vi "dfd_FXP Lattice ARMA (normalized) with IS.vi"(6 "state in":i64[](array[numeric]), 7 "FXPOPs":T5[](array[typedef]) {"source" items=["Coef a/k"=0, "Coef b/v"=7, "Input"=1, "Output"=2, "Multiplicand"=3, "Product"=4, "Sum"=5, "Delay"=6, "Gain"=8]}, 8 "filtering statistics in":T4(array[cluster]) {"statistics information"."min value" format="%.2f"; "statistics information"."max value" format="%.2f"; "Quantizer Source" items=["Coefficients a/k"=0, "Coefficients b/v"=7, "Input"=1, "Output"=2, "Multiplicand"=3, "Product"=4, "Sum"=5, "Delay"=6]}, 9 "coef v":T7, 10 "coef k & ^k":T7, 11 "X":T7) -> (0 "filtering statistics out":T4(array[cluster]) {"statistics information"."min value" format="%.2f"; "statistics information"."max value" format="%.2f"; "Quantizer Source" items=["Coefficients a/k"=0, "Coefficients b/v"=7, "Input"=1, "Output"=2, "Multiplicand"=3, "Product"=4, "Sum"=5, "Delay"=6]}, 3 "filtered X":T7, 4 "state out":i64[](array[numeric]))   [LabVIEW 2017, in "NI_DigFilter_FXP.lvlib"]
uses:
  <vilib>/addons/Digital Filter Design/NI_DigFilter_FXP.lvlib
  <vilib>/addons/Digital Filter Design/_Objects.llb/dfd_DFXP Data Type (vector).ctl
  <vilib>/addons/Digital Filter Design/_Objects.llb/dfd_DFXP Operation Parameter.ctl
  <vilib>/addons/Digital Filter Design/_Objects.llb/dfd_Internal Quantization Srcs.ctl
  <vilib>/addons/Digital Filter Design/_Objects.llb/DFD Quantization Sources.ctl
  <vilib>/addons/Digital Filter Design/_Objects.llb/DFD FXP Statistics Data.ctl
  <vilib>/addons/Digital Filter Design/_Objects.llb/dfd_DFXP Data Type (scaler).ctl
  <vilib>/addons/Digital Filter Design/NI_DigFilterLicensed.lvlib
panel:
  in  "DFXP Value":T1={"value"=0, "wl"=0, "iwl"=0, "Signed"=TRUE} {"value" format="%.0x"}
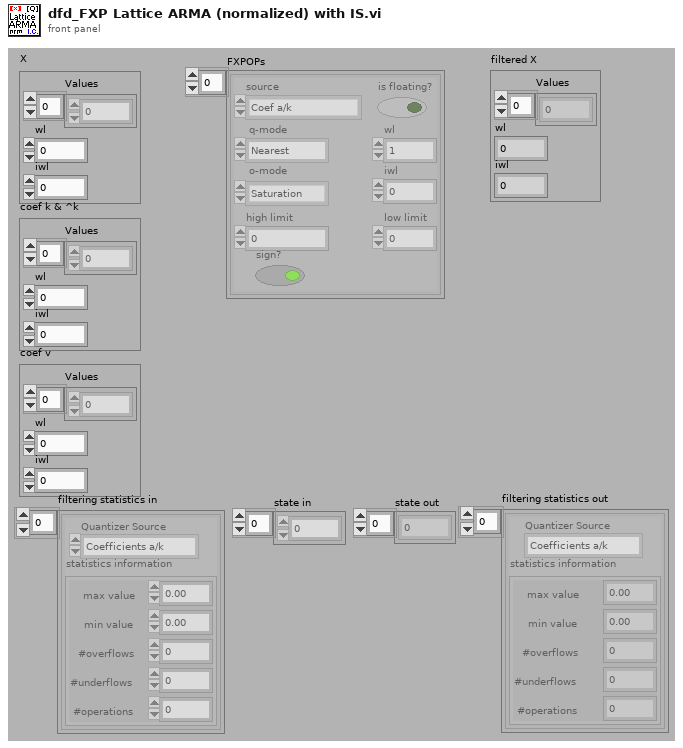
[diagram p1: front panel]
types:
  T1 = typedef "dfd_DFXP Data Type (scaler).ctl" = cluster{"value":i64, "wl":i16, "iwl":i16, "Signed":bool}
  T2 = typedef "NI_DigFilterLicensed.lvlib/DFD Quantization Sources.ctl" = u16
  T3 = typedef "NI_DigFilterLicensed.lvlib/DFD FXP Statistics Data.ctl" = cluster{"max value":ext, "min value":ext, "#overflows":i32, "#underflows":i32, "#operations":i32}
  T4 = cluster{"Quantizer Source":T2, "statistics information":T3}[]
  T5 = typedef "dfd_DFXP Operation Parameter.ctl" = cluster{"source":T6, "is floating?":bool, "o-mode":enum16{"Saturation", "Wrap"}, "q-mode":enum16{"Nearest", "Truncation"}, "wl":i16, "high limit":i64, "low limit":i64, "iwl":i16, "sign?":bool}
  T6 = typedef "NI_DigFilterLicensed.lvlib/dfd_Internal Quantization Srcs.ctl" = u16
  T7 = typedef "dfd_DFXP Data Type (vector).ctl" = cluster{"Values":i64[], "wl":i16, "iwl":i16}
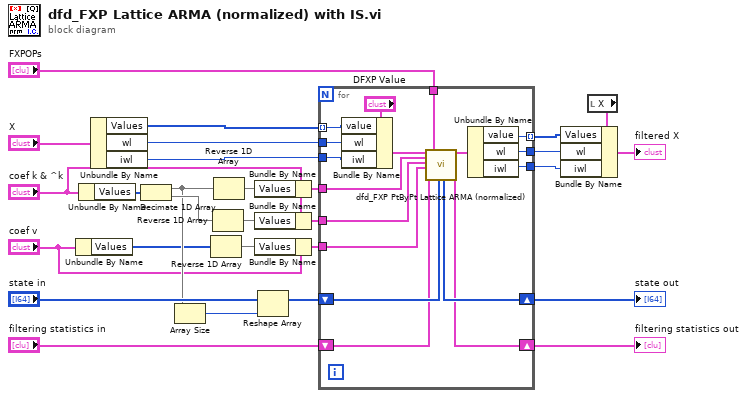
[diagram p0: block diagram]
diagram:
  n1 = Unbundle By Name("coef v") -> ("Values"=w13:i64[])
  n2 = Unbundle By Name("coef k & ^k") -> ("Values"=w14:i64[])
  n3 = Unbundle By Name("X") -> ("Values"=w7:i64[], "wl"=w6:i16, "iwl"=w5:i16)
  n4 = Decimate 1D Array(w14) -> (w26:i64[], w27:i64[])
  n5 = Array Size(array=w26) -> (size(s)=w20:i32)
  n6 = Reverse 1D Array(array=w13) -> (reversed array=w19:i64[])
  n7 = Reverse 1D Array(array=w27) -> (reversed array=w22:i64[])
  n8 = Reverse 1D Array(array=w26) -> (reversed array=w25:i64[])
  n9 = Bundle By Name(cluster="coef k & ^k", "Values"=w25) -> (w12:T7)
  n10 = Bundle By Name(cluster="coef k & ^k", "Values"=w22) -> (w11:T7)
  n11 = Bundle By Name(cluster="coef v", "Values"=w19) -> (w9:T7)
  n12 = Reshape Array("state in", w20) -> (w23:i64[])
  n13 = for {
    tunnel: w7 -> [w45] mode=indexing
    tunnel: w12 -> [w44]
    shift-right: [w40] -> w21
    shift-left: w23 -> [w41]
    tunnel: w11 -> [w43]
    tunnel: w9 -> [w42]
    tunnel: [w31] -> w18 mode=indexing
    tunnel: "FXPOPs" -> [w38]
    shift-right: [w36] -> w15
    shift-left: "filtering statistics in" -> [w37]
    tunnel: w6 -> [w33]
    tunnel: w5 -> [w32]
    tunnel: [w30] -> w2
    tunnel: [w29] -> w1
    n14 = Bundle By Name(cluster="DFXP Value", "value"=w45, "wl"=w33, "iwl"=w32) -> (w35:T1)
    n15 = call <vilib>:"dfd_FXP PtByPt Lattice ARMA (normalized).vi"("x"=w35, "coef k[M..1]"=w44, "coef ^k[M..1]"=w43, "coef v[M..0]"=w42, "filtering statistics in"=w37, "FXPOPs"=w38, "state in"=w41) -> ("state out"=w40:i64[], "filtered x"=w39:T1, "filtering statistics out"=w36:T4)  [unwired: 10 out]
    n16 = Unbundle By Name(w39) -> ("value"=w31:i64, "wl"=w30:i16, "iwl"=w29:i16)
  }
  "state out" <- w21
  "filtering statistics out" <- w15
  n17 = local read "X"() -> (w3:T7)
  n18 = Bundle By Name(cluster=w3, "Values"=w18, "wl"=w2, "iwl"=w1) -> (→"filtered X":T7)
